vi "Check data length TCP 0.vi"(11 "# samples in buffer":u16) -> (2 "Modbus Function":T1, 3 "# samples in buffer out":u16)   [LabVIEW 2022 SP3]
uses:
  Ctl/Modbus Function TCP.ctl
panel:
  in  "bulk mode trigger (size)":u16=1230
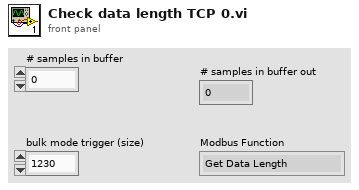
[diagram p1: front panel]
types:
  T1 = typedef "Modbus Function TCP.ctl" = enum16{"Get Data Length", "Normal Mode", "Bulk Mode", "Reconnect Port", "Recconect Box"}
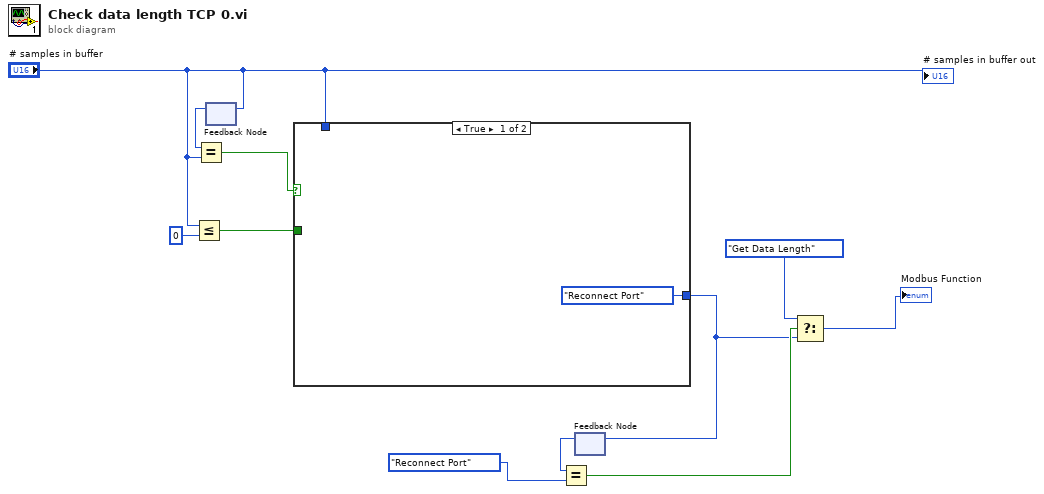
[diagram p0: block diagram]
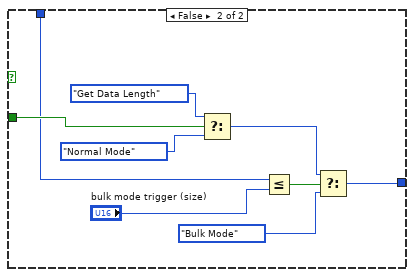
[diagram p2: hidden frame]
diagram:
  n1 = Less Or Equal?(x="# samples in buffer", y=u16 0) -> (x <= y?=w10:bool)
  n2 = feedback-in #1("# samples in buffer") -> ()
  n3 = feedback #1() -> (w9:u16)  [unwired: 1 in]
  n4 = Equal?(x=w9, y="# samples in buffer") -> (x = y?=w7:bool)
  n5 = case shown="True" w7 {
    tunnel: w10 -> [_ w21]
    tunnel: [Modbus_Function_TCP."Reconnect Port" ("Modbus") w17] -> w2
    tunnel: "# samples in buffer" -> [_ w13]
    frame True {
    }
    frame False {
      n6 = Select(t=Modbus_Function_TCP."Get Data Length" ("Modbus"), s=w21, f=Modbus_Function_TCP."Normal Mode" ("Modbus")) -> (s? t:f=w19:T1)
      n7 = Less Or Equal?(x=w13, y="bulk mode trigger (size)") -> (x <= y?=w20:bool)
      n8 = Select(t=w19, s=w20, f=Modbus_Function_TCP."Bulk Mode" ("Modbus")) -> (s? t:f=w17:T1)
    }
  }
  n9 = feedback #2() -> (w6:T1)  [unwired: 1 in]
  n10 = Equal?(x=w6, y=Modbus_Function_TCP."Reconnect Port" ("Modbus")) -> (x = y?=w4:bool)
  n11 = feedback-in #2(w2) -> ()
  n12 = Select(t=Modbus_Function_TCP."Get Data Length" ("Modbus"), s=w4, f=w2) -> (s? t:f=→"Modbus Function":T1)
  "# samples in buffer out" <- "# samples in buffer"
